vi "Read U8 From 1 Address.vi"(8 "Error in (no error)":errorcluster, 9 "Address number (0)":u8 max=49, 10 "Motor ID (0)":u8, 11 "VISA resource name":refnum<visa-resource-name>) -> (0 "error out":errorcluster, 2 "Data":u8, 3 "VISA resource name out":refnum<visa-resource-name>)   [LabVIEW 2016, in "Dynamixel Motor.lvlib"]
doc: "Reads a single value/address from the motor's register. This is a Low-Level VI that is used by other VIs."
uses:
  Dynamixel Motor.lvlib
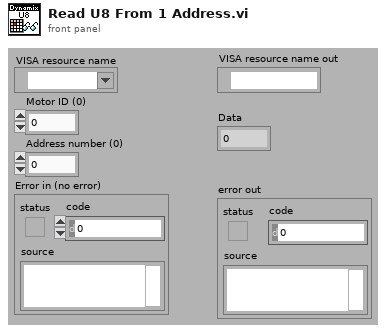
[diagram p1: front panel]
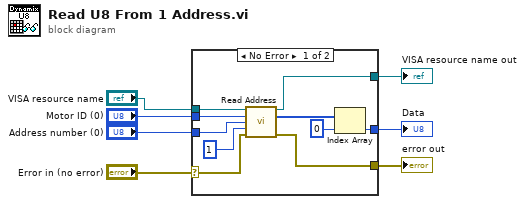
[diagram p0: block diagram]
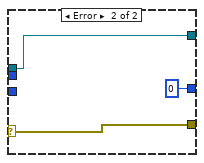
[diagram p2: hidden frame]
diagram:
  n1 = case shown="No Error" "Error in (no error)" {
    selector: "Error in (no error)" -> [w8 w19]
    tunnel: [w17 u8 0 ("Numeric")] -> w7
    tunnel: "VISA resource name" -> [w14 w20]
    tunnel: [w13 w20] -> w5
    tunnel: [w12 w19] -> w4
    tunnel: "Motor ID (0)" -> [w10 _]
    tunnel: "Address number (0)" -> [w9 _]
    frame No Error {
      n2 = call "Read Address.vi"("VISA resource name"=w14, "Motor ID (0)"=w10, "Address number (0)"=w9, "Number of Addresses to read (1)"=u8 1, "Error in (no error)"=w8) -> ("VISA resource name Out"=w13:refnum<visa-resource-name>, "Data Read"=w15:u8[], "error out"=w12:errorcluster)  [unwired: 7 in, 1 out]
      n3 = Index Array(array=w15, index=0) -> (element=w17:u8)
    }
    frame Error {
    }
  }
  "Data" <- w7
  "VISA resource name out" <- w5
  "error out" <- w4
